vi "Update.vi"(8 "error in (no error)":errorcluster, 11 "senseHatDisplay in":refnum<class "RPI.SenseHat.Display.lvclass">) -> (0 "error out":errorcluster, 3 "senseHatDisplay out":refnum<class "RPI.SenseHat.Display.lvclass">)   [LabVIEW 2020, in "RPI.SenseHat.Display.lvlib" / "RPI.SenseHat.Display.lvclass"]
doc: "Copies the colors in the Screen property array to the physical Sense HAT display."
uses:
  RPI.SenseHat.Display.lvclass
  RPI.SenseHat.Display.lvclass/RPI.SenseHat.Display.ctl
  Pixel/Pixel.lvclass
  Image/Image.lvclass
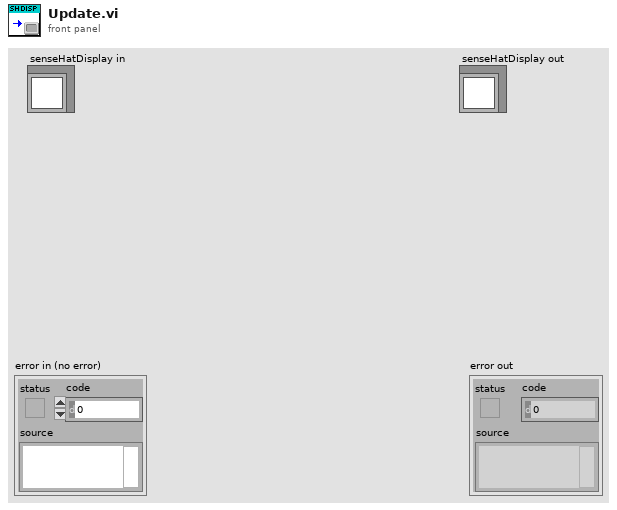
[diagram p1: front panel]
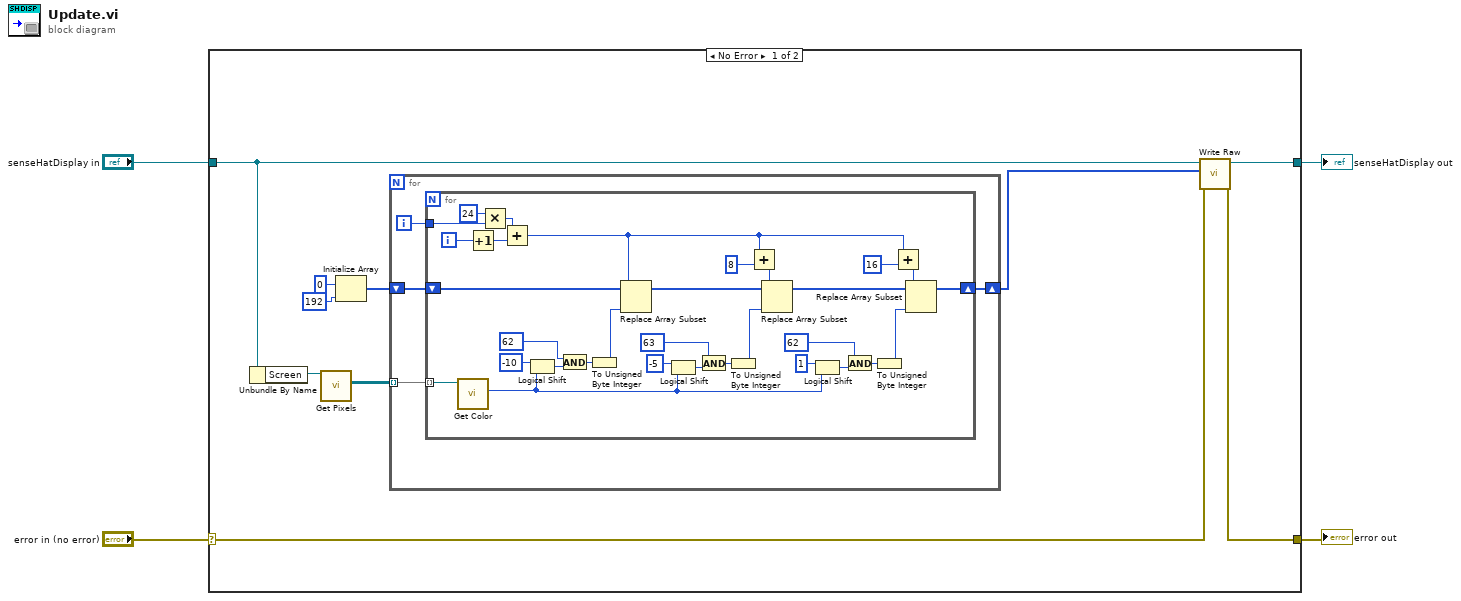
[diagram p0: block diagram]
diagram:
  n1 = case shown="No Error" "error in (no error)" {
    selector: "error in (no error)" -> [w13 w51]
    tunnel: [w12 w51] -> w3
    tunnel: [w14 w50] -> w1
    tunnel: "senseHatDisplay in" -> [w11 w50]
    frame No Error {
      n2 = Unbundle By Name(w11) -> ("Screen"=w10:refnum<class "Image.lvclass">)
      n3 = call "Get Pixels.vi"("Image in"=w10) -> ("Pixels"=w9:refnum<class "Pixel.lvclass">[][])  [unwired: 8 in, 2 out]
      n4 = Initialize Array(u8 0 ("element"), 192 ("dimension size")) -> (w6:u8[])
      n5 = for {
        tunnel: w9 -> [w18] mode=indexing
        shift-right: [w16] -> w5
        shift-left: w6 -> [w17]
        i -> [w15]
        n6 = for {
          tunnel: w18 -> [w49] mode=indexing
          shift-right: [w42] -> w16
          shift-left: w17 -> [w48]
          tunnel: w15 -> [w45]
          i -> [w20]
          n7 = call-dynamic "Get Color.vi"("Pixel in"=w49) -> ("Color"=w23:u16)  [unwired: 8 in, 2 out]
          n8 = Increment(x=w20) -> (x+1=w19:i32)
          n9 = Multiply(x=24, y=w45) -> (x*y=w47:i32)
          n10 = Add(x=w47, y=w19) -> (x+y=w21:i32)
          n11 = Logical Shift(y=i16 -10, x=w23) -> (x << y=w37:u16)
          n12 = And(x=u16 62, y=w37) -> (x .and. y?=w36:u16)
          n13 = To Unsigned Byte Integer(number=w36) -> (unsigned 8bit integer=w33:u8)
          n14 = Replace Array Subset(array=w48, new element=w33, index=w21) -> (w44:u8[])
          n15 = Logical Shift(y=i16 -5, x=w23) -> (x << y=w31:u16)
          n16 = And(x=u16 63, y=w31) -> (x .and. y?=w30:u16)
          n17 = To Unsigned Byte Integer(number=w30) -> (unsigned 8bit integer=w28:u8)
          n18 = Add(x=w21, y=8) -> (x+y=w39:i32)
          n19 = Replace Array Subset(array=w44, new element=w28, index=w39) -> (w43:u8[])
          n20 = Logical Shift(y=i16 1, x=w23) -> (x << y=w26:u16)
          n21 = And(x=u16 62, y=w26) -> (x .and. y?=w25:u16)
          n22 = To Unsigned Byte Integer(number=w25) -> (unsigned 8bit integer=w22:u8)
          n23 = Add(x=w21, y=16) -> (x+y=w38:i32)
          n24 = Replace Array Subset(array=w43, new element=w22, index=w38) -> (w42:u8[])
        }
      }
      n25 = call "Write Raw.vi"("error in (no error)"=w13, "Data"=w5, "senseHatDisplay in"=w11) -> ("error out"=w12:errorcluster, "senseHatDisplay out"=w14:refnum<class "RPI.SenseHat.Display.lvclass">)  [unwired: 7 in]
    }
    frame Error {
    }
  }
  "error out" <- w3
  "senseHatDisplay out" <- w1
